vi "Read Enable.vi"(8 "error in (no error)":errorcluster, 11 "CsvReportPlugin in":refnum<class "CsvReportPlugin.lvclass">) -> (0 "error out":errorcluster, 2 "Enable":bool, 3 "CsvReportPlugin out":refnum<class "CsvReportPlugin.lvclass">)   [LabVIEW 2015, in "CsvReportPlugin.lvclass"]
uses:
  CsvReportPlugin.lvclass
  CsvReportPlugin.lvclass/CsvReportPlugin.ctl
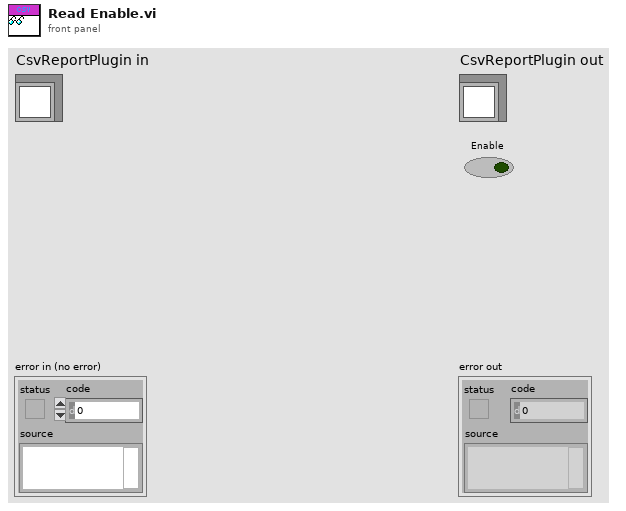
[diagram p1: front panel]
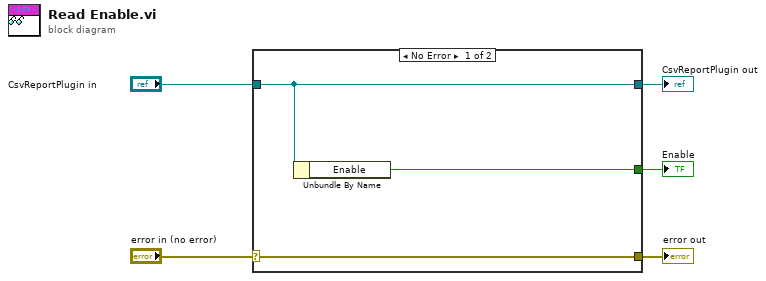
[diagram p0: block diagram]
diagram:
  n1 = case shown="No Error" "error in (no error)" {
    selector: "error in (no error)" -> [w8 w9]
    tunnel: [w8 w9] -> w4
    tunnel: [w7 w10] -> w2
    tunnel: "CsvReportPlugin in" -> [w7 w10]
    tunnel: [w6 _] -> w1
    frame No Error {
      n2 = Unbundle By Name(w7) -> ("Enable"=w6:bool)
    }
    frame Error {
    }
  }
  "error out" <- w4
  "CsvReportPlugin out" <- w2
  "Enable" <- w1
